vi "Demo Sensor Read.vi"() -> ()   [LabVIEW 2012]
doc: "The Basic Serial Read and Write example performs a Serial Port Read, a Serial Port Write, or a combination of these actions. The user selects the actions (read or write) on the front panel. If both are selected, the VI will write the data first, read data, and then close the VISA session that is opened to the port. This VI will wait until the specified number of bytes is received at the port. Only the number of bytes specified will be read.\n\nINSTRUCTIONS:\n1) Select the serial resource and configuration parameters (baud rate, data bits, parity, stop bits, flow control).\n2) Select the operations to be performed. \n3) Connect the serial port to your device. If no device is available, perform a loopback test by doing one of the following. Short pins 2 and 3 on a RS-232 cable or short pin 4 to pin 8 and pin 5 to pin 9 on a RS-485/422 cable. \n4) Run the VI to see the data read. (The \"read string\" will match the \"string to write\" if a loopback test was performed.)\n\nNote: The parameters set for the serial port must match the parameters of the connected instrument or device. In this example, the bytes to read parameter specifies the number of bytes that the serial port reads. If there were more bytes at the port than the number specified in bytes to read, those bytes would not be read. Also, if you specify to read more bytes than the number of bytes actually read, you might receive a timeout error message.\n\nOn the block diagram, the Configure Serial Port VI sets the configuration parameters. The front panel displays the controls used to configure the basic parameters, such as baud rate, data bits, and parity. Constants configure the other parameters the user probably does not need set. After the VISA Configure Serial Port VI opens the VISA session and configures the port, the VI passes the VISA resource name to other VIs that perform operations on that VISA resource. The VISA Write function sends a command to the serial device and the VISA Read function returns data based on the command. The VISA Close function then closes the reference to the serial device. It is important to close the reference; otherwise communication through with that port through protocols other than VISA might not be possible."
uses:
  12bit_2sComplement_array.vi
panel:
  in  "Accel Range":dbl
  out "decimated array":dbl[](array[numeric]) format="%.6f"
  in  "ByteArray in":u8[](array[numeric]) format="%b"
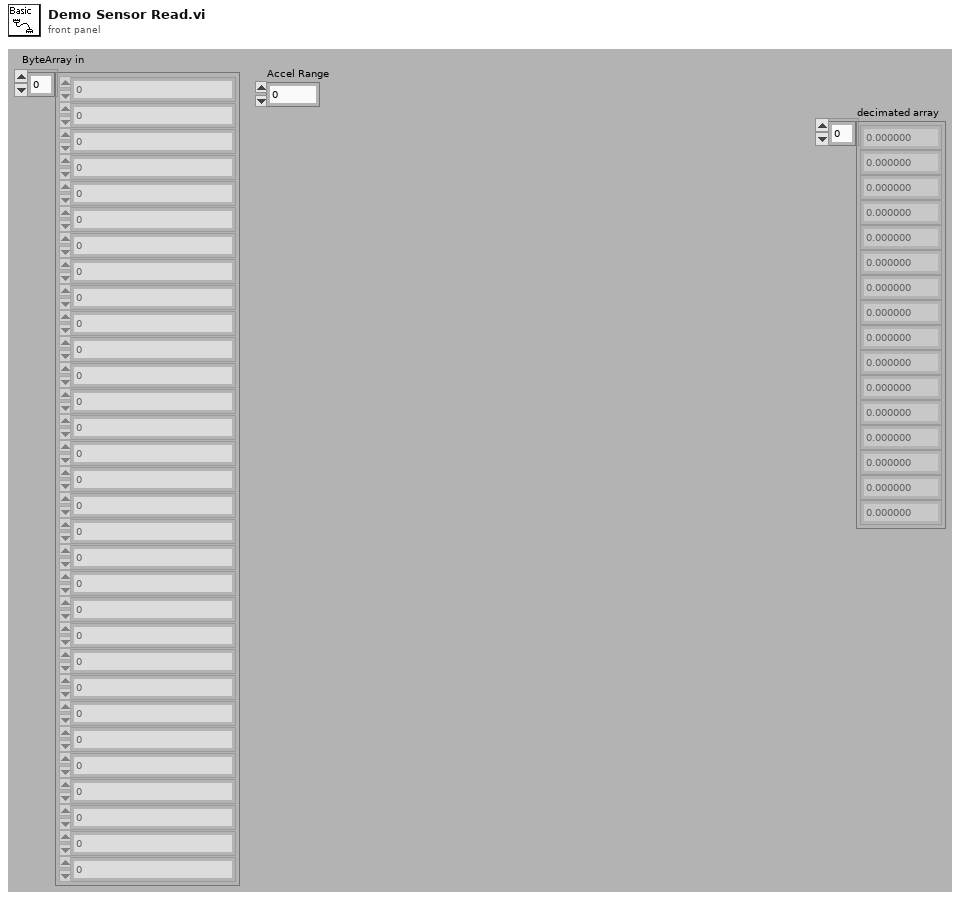
[diagram p1: front panel]
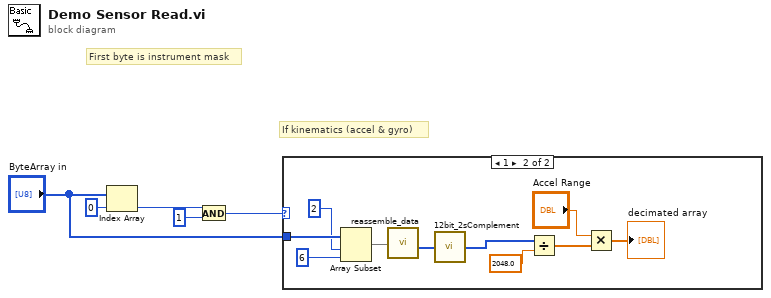
[diagram p0: block diagram]
diagram:
  # "If kinematics (accel & gyro)"
  # "First byte is instrument mask"
  n1 = Index Array(array="ByteArray in", index=0) -> (element=w4:u8)
  n2 = And(x=w4, y=u8 1) -> (x .and. y?=w2:u8)
  n3 = case shown="1" w2 {
    tunnel: "ByteArray in" -> [_ w15]
    frame 0, Default {
    }
    frame 1 {
      n4 = Array Subset(array=w15, index=2, length=6) -> (w12:u8[])
      n5 = call "reassemble_data.vi"("Interleaved 8bit Array"=w12) -> ("reassembled 16 bit"=w10:u16[])  [unwired: 8 in, 2 out]
      n6 = call-poly "12bit_2sComplement.vi"("binary"=w10) -> ("decimal"=w8:i16[])
      n7 = Divide(x=w8, y=2048.0 ("Decimal")) -> (x/y=w7:dbl[])
      n8 = Multiply(x="Accel Range", y=w7) -> (x*y=→"decimated array":dbl[])
    }
  }
